vi "Gear Line Up - Copy.vi"(4 "R/G/B":cluster{"Lower value":i32, "Upper value":i32}[](array[cluster])=[{"Lower value"=0, "Upper value"=40}, {"Lower value"=80, "Upper value"=255}, {"Lower value"=0, "Upper value"=255}], 5 "Camera Image":T1, 6 "Angle Reduction Factor":dbl, 8 "Error in":errorcluster) -> (0 "Error out":errorcluster, 2 "Right Output":dbl, 3 "Left Output":dbl)   [LabVIEW 2016]
uses:
  <vilib>/vision/Image Controls.llb/IMAQ Image.ctl
panel:
  out "Image Dimensions":cluster{"X Resolution":i32, "Y Resolution":i32}
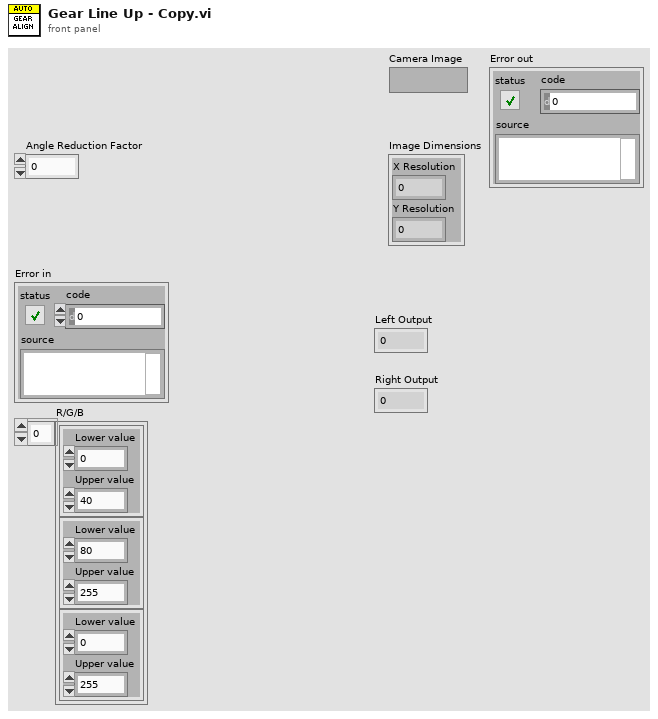
[diagram p1: front panel]
types:
  T1 = typedef "IMAQ Image.ctl" = refnum<image>
  T2 = cluster{"Left":dbl, "Top":dbl, "Right":dbl, "Bottom":dbl}
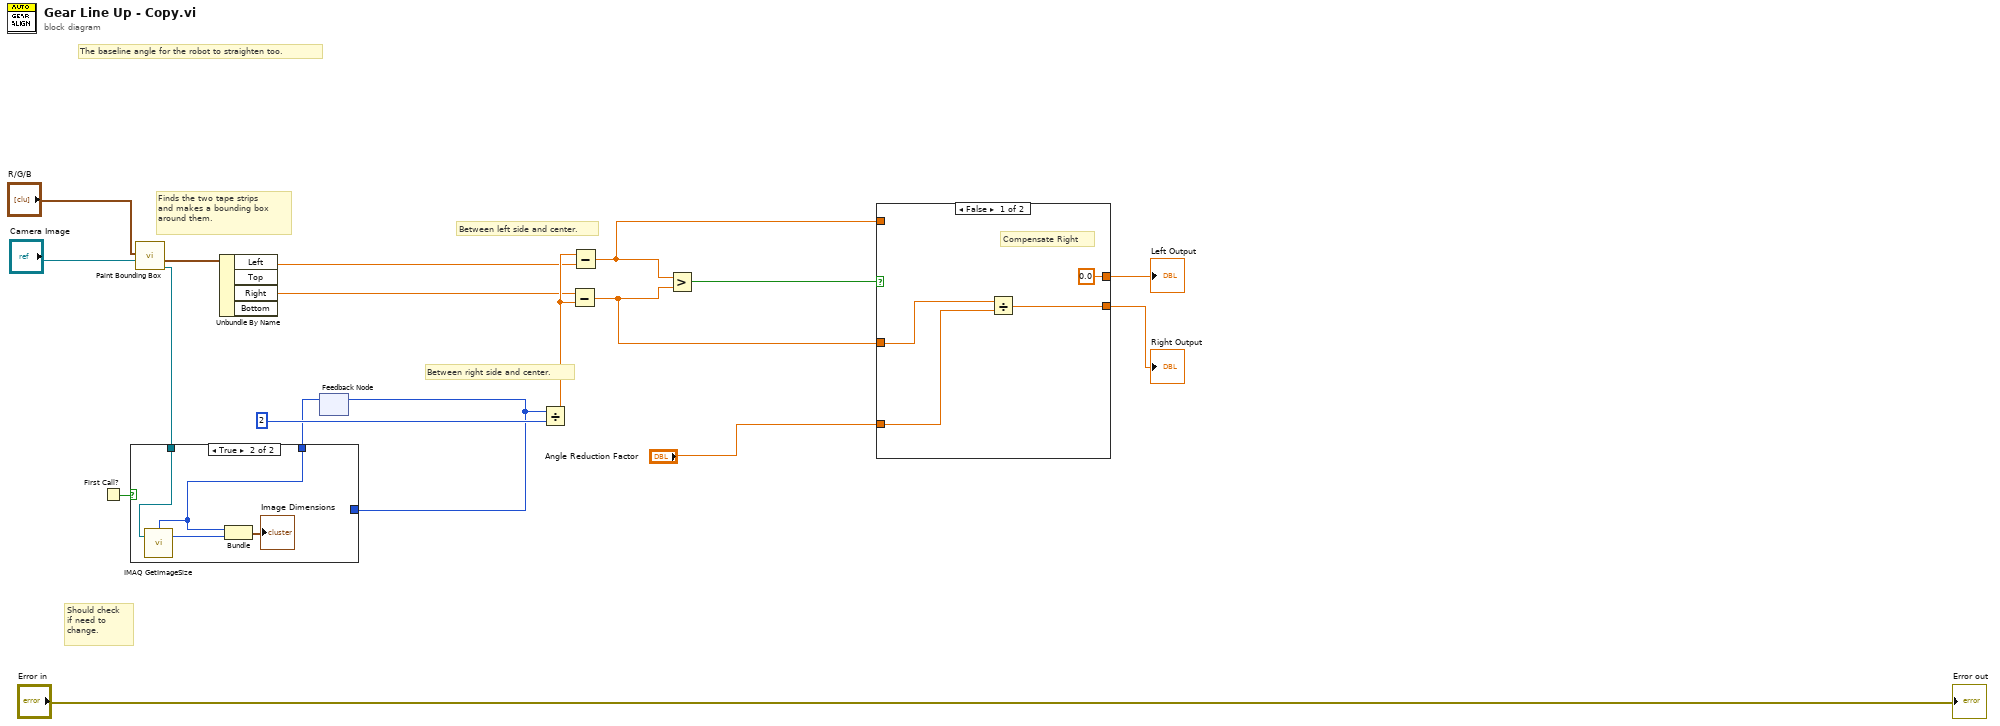
[diagram p0: block diagram]
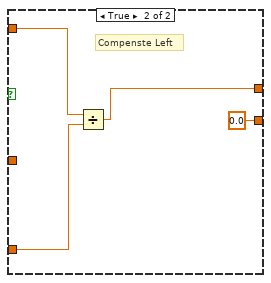
[diagram p2: hidden frame]
diagram:
  # "Between right side and center."
  # "Between left side and center."
  # "Finds the two tape strips\nand makes a bounding box\naround them."
  # "The baseline angle for the robot to straighten too."
  # "Should check\nif need to\nchange."
  n1 = First Call?() -> (First Call?: T/F=w13:bool)
  n2 = call "Paint Bounding Box.vi"("Camera Image"="Camera Image", "R/G/B"="R/G/B") -> ("Thresholded Image"=w12:T1, "Bounding Box Final"=w15:T2)  [unwired: 5 in, 3 out]
  n3 = Unbundle By Name(w15) -> ("Left"=w2:dbl, "Right"=w3:dbl)  [unwired: 2 out]
  n4 = feedback #1() -> (w10:i32)  [unwired: 1 in]
  n5 = case shown="True" w13 {
    tunnel: [w19 w21] -> w11
    tunnel: w12 -> [_ w20]
    tunnel: w10 -> [w19 _]
    frame False {
    }
    frame True {
      n6 = call "IMAQ GetImageSize"("Image"=w20) -> ("Y Resolution"=w22:i32, "X Resolution"=w21:i32)  [unwired: 3 in, 1 out]
      n7 = Bundle("X Resolution"=w21, "Y Resolution"=w22) -> (→"Image Dimensions":cluster{"X Resolution":i32, "Y Resolution":i32})  [unwired: 1 in]
    }
  }
  n8 = feedback-in #1(w11) -> ()
  n9 = Divide(x=w10, y=2) -> (x/y=w9:dbl)
  n10 = Subtract(x=w3, y=w9) -> (x-y=w7:dbl)
  n11 = Subtract(x=w9, y=w2) -> (x-y=w8:dbl)
  n12 = Greater?(x=w8, y=w7) -> (0:w6:bool)
  n13 = case shown="False" w6 {
    tunnel: w8 -> [_ w31]
    tunnel: "Angle Reduction Factor" -> [w27 w30]
    tunnel: w7 -> [w26 _]
    tunnel: [w25 0.0] -> w5
    tunnel: [0.0 w29] -> w4
    frame False {
      # "Compensate Right"
      n14 = Divide(x=w26, y=w27) -> (x/y=w25:dbl)
    }
    frame True {
      # "Compenste Left"
      n15 = Divide(x=w31, y=w30) -> (x/y=w29:dbl)
    }
  }
  "Left Output" <- w4
  "Right Output" <- w5
  "Error out" <- "Error in"
